vi "Remove Multibyte Characters.vi"(8 "error in (no error)":errorcluster, 11 "String":string) -> (0 "error out":errorcluster, 2 "Any Multibyte Removed?":bool, 3 "String with Multibyte Removed":string)   [LabVIEW 2017, in "NI_Multibyte Utilities.lvlib"]
uses:
  <vilib>/Utility/Multibyte/NI_Multibyte Utilities.lvlib
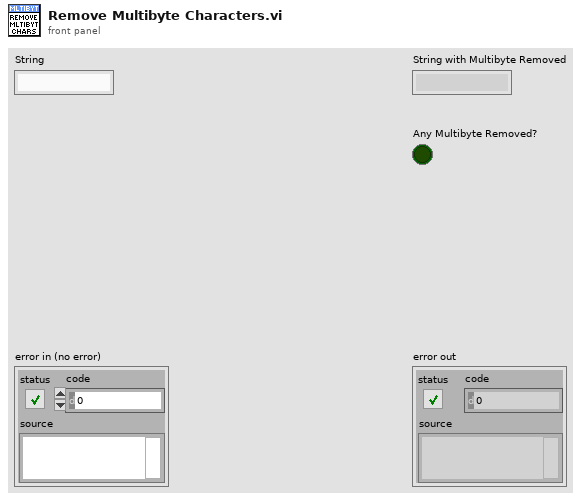
[diagram p1: front panel]
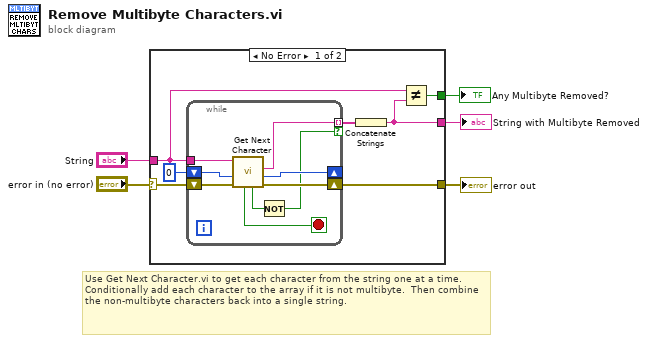
[diagram p0: block diagram]
diagram:
  # "Use Get Next Character.vi to get each character from the string one at a time. Conditionally add each character to the array if it is not multibyte.  Then combine the non-multibyte characters back into a single string."
  n1 = case shown="No Error" "error in (no error)" {
    selector: "error in (no error)" -> [w10 w22]
    tunnel: "String" -> [w8 _]
    tunnel: [w7 _] -> w4
    tunnel: [w9 w22] -> w2
    tunnel: [w6 _] -> w1
    frame No Error {
      n2 = while {
        shift-right: [w20] -> w9
        shift-left: w10 -> [w21]
        shift-right: [w18] -> _
        shift-left: 0 -> [w19]
        tunnel: w8 -> [w16]
        tunnel: [w13] -> w11 mode=indexing if=w14
        stop <- w17 stop-if-true
        n3 = call <vilib>:"Get Next Character.vi"("error in (no error)"=w21, "Offset in"=w19, "String"=w16) -> ("error out"=w20:errorcluster, "Offset out"=w18:i32, "Character"=w13:string, "Multibyte?"=w15:bool, "Past End of String?"=w17:bool)  [unwired: 3 in, 1 out]
        n4 = Not(x=w15) -> (.not. x?=w14:bool)
      }
      n5 = Concatenate Strings(w11) -> (w7:string)
      n6 = Not Equal?(x=w8, y=w7) -> (x != y?=w6:bool)
    }
    frame Error {
    }
  }
  "error out" <- w2
  "String with Multibyte Removed" <- w4
  "Any Multibyte Removed?" <- w1
